vi "DS18B20 Master VI.vi"(6 "Reset Delay (ms)":u32=100, 7 "1-Wire DIO Pin":refnum<k21>="ConnectorA/DIO15", 8 "error in":errorcluster, 9 "Master Function Command":T1, 10 "ROM Command":T2=enum."Skip ROM Command") -> (0 "error out":errorcluster, 1 "Scratchpad Data":u8[](array[numeric]) format="%.0x", 2 "ROM Data":u8[](array[numeric]) format="%.0x", 4 "Convert Time (usec)":u32, 5 "Supply Mode":bool)   [LabVIEW 2014]
uses:
  ROM Commands.ctl
  Master Function Commands.ctl
  <vilib>/rvi/Emulation/niFpgaGetClockAttributes.vi
  <vilib>/rvi/Emulation/niFpgaSctlEmulationGetInTimedLoop.vi
  <vilib>/rvi/Emulation/niFpgaEmulationReportErrorSimple.vi
  <vilib>/rvi/Emulation/niFpgaCriticalErrorInLSC.vi
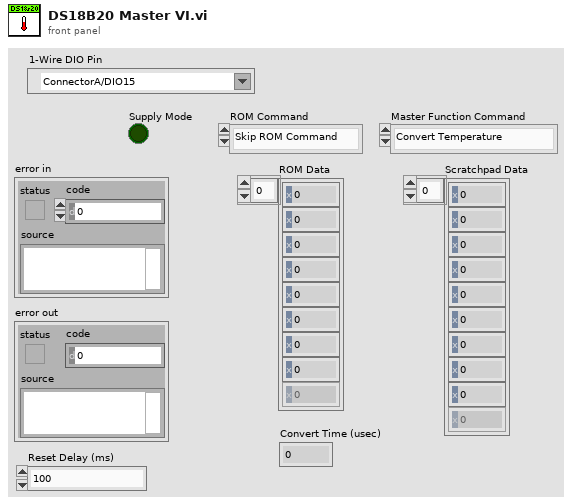
[diagram p1: front panel]
types:
  T1 = typedef "Master Function Commands.ctl" = enum16{"Convert Temperature", "Read Scratchpad", "Read Power Supply"}
  T2 = typedef "ROM Commands.ctl" = enum16{"Read ROM", "Skip ROM Command"}
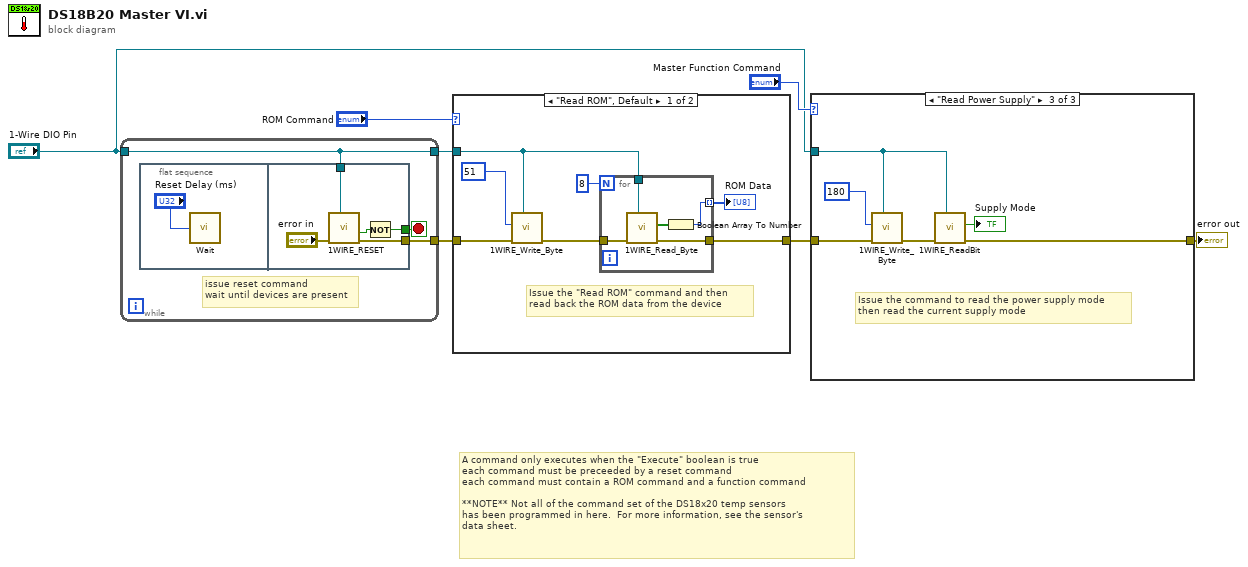
[diagram p0: block diagram]
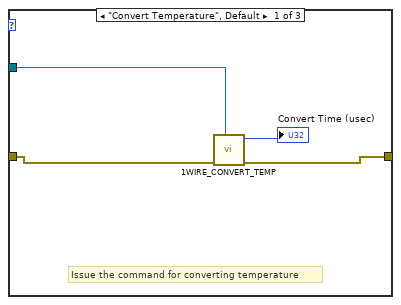
[diagram p2: hidden frame]
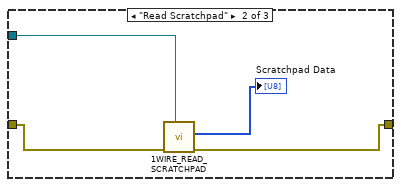
[diagram p3: hidden frame]
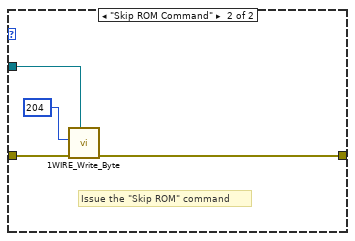
[diagram p4: hidden frame]
diagram:
  # "A command only executes when the \"Execute\" boolean is true\neach command must be preceeded by a reset command\neach command must contain a ROM command and a function command\n\n**NOTE** Not all of the command set of the DS18x20 temp sensors\nhas been programmed in here.  For more information, see the sensor's\ndata sheet."
  n1 = while {
    tunnel: [w9] -> w5
    tunnel: "1-Wire DIO Pin" -> [w8]
    tunnel: [w8] -> w2
    stop <- w10 stop-if-true
    # "issue reset command\nwait until devices are present"
    n2 = flat-sequence {
      tunnel: [w15] -> w10
      tunnel: [w14] -> w9
      tunnel: w8 -> [w12]
      frame #0 {
        n3 = call "Wait"("Count(mSec)"="Reset Delay (ms)") -> ()  [unwired: 1 out]
      }
      frame #1 {
        n4 = call "1WIRE_RESET.vi"("1-Wire DIO Pin"=w12, "error in"="error in") -> ("error out"=w14:errorcluster, "0 = Device Present / 1=no"=w13:bool)  [unwired: 8 in]
        n5 = Not(x=w13) -> (.not. x?=w15:bool)
      }
    }
  }
  n6 = case shown="\"Read ROM\", Default" "ROM Command" {
    tunnel: w5 -> [w21 w32]
    tunnel: [w19 w31] -> w4
    tunnel: w2 -> [w17 w29]
    frame "Read ROM", Default {
      # "Issue the \"Read ROM\" command and then\nread back the ROM data from the device"
      n7 = call "1WIRE_Write_Byte.vi"("1-Wire DIO Pin"=w17, "error in"=w21, "Tx data"=u8 51 ("Tx data 2")) -> ("error out"=w23:errorcluster)  [unwired: 7 in, 1 out]
      n8 = for {
        N: 8 -> [_]
        tunnel: w23 -> [w28]
        tunnel: [w27] -> w19
        tunnel: [w25] -> w20 mode=indexing
        tunnel: w17 -> [w24]
        n9 = call "1WIRE_Read_Byte.vi"("1-Wire DIO Pin"=w24, "error in"=w28) -> ("error out"=w27:errorcluster, "Array"=w26:bool[])  [unwired: 8 in]
        n10 = Boolean Array To Number(Boolean array=w26) -> (number=w25:u8)
      }
      "ROM Data" <- w20
    }
    frame "Skip ROM Command" {
      # "Issue the \"Skip ROM\" command"
      n11 = call "1WIRE_Write_Byte.vi"("1-Wire DIO Pin"=w29, "error in"=w32, "Tx data"=u8 204) -> ("error out"=w31:errorcluster)  [unwired: 7 in, 1 out]
    }
  }
  n12 = case shown="\"Read Power Supply\"" "Master Function Command" {
    tunnel: w4 -> [w36 w40 w45]
    tunnel: [w35 w39 w43] -> w6
    tunnel: "1-Wire DIO Pin" -> [w33 w37 w41]
    frame "Convert Temperature", Default {
      # "Issue the command for converting temperature"
      n13 = call "1WIRE_CONVERT_TEMP.vi"("1-Wire DIO Pin"=w33, "error in (no error)"=w36) -> ("error out"=w35:errorcluster, "Convert Time (usec)"=→"Convert Time (usec)":u32)  [unwired: 8 in]
    }
    frame "Read Scratchpad" {
      n14 = call "1WIRE_READ_SCRATCHPAD.vi"("1-Wire DIO Pin"=w37, "error in (no error)"=w40) -> ("error out"=w39:errorcluster, "Scratchpad Data"=→"Scratchpad Data":u8[])  [unwired: 7 in]
    }
    frame "Read Power Supply" {
      # "Issue the command to read the power supply mode\nthen read the current supply mode"
      n15 = call "1WIRE_Write_Byte.vi"("1-Wire DIO Pin"=w41, "error in"=w45, "Tx data"=u8 180 ("Tx data 2")) -> ("error out"=w44:errorcluster)  [unwired: 7 in, 1 out]
      n16 = call "1WIRE_ReadBit.vi"("1-Wire DIO Pin"=w41, "error in"=w44) -> ("error out"=w43:errorcluster, "Bit Read"=→"Supply Mode":bool)  [unwired: 8 in]
    }
  }
  "error out" <- w6
